vi "FPGAcode.vi"() -> ()   [LabVIEW 2015]
uses:
  <vilib>/Platform/TimedLoop/XDataNode/timing_clust.ctl
  <vilib>/Platform/TimedLoop/XDataNode/nitl_modes.ctl
  <vilib>/Platform/TimedLoop/XDataNode/wakeup.ctl
  <vilib>/rvi/Emulation/niFpgaGetClockAttributes.vi
  <vilib>/rvi/Emulation/niFpgaSctlEmulationGetInTimedLoop.vi
  <vilib>/rvi/Emulation/niFpgaEmulationReportErrorSimple.vi
  <vilib>/rvi/Emulation/niFpgaProcessEmulError.vi
  <vilib>/rvi/eio/common/nirviEmuTemplateMethod_errors.vi
  <vilib>/rvi/Emulation/niFpgaCriticalErrorInLSC.vi
  <vilib>/eio/EIONode/EIONode.xnode
  <vilib>/Platform/TimedLoop/XDataNode/XDataNode.xnode
  <vilib>/Platform/TimedLoop/XDataNode/XDNodeRunTimeDep.lvlib
panel:
  in  "User Command Commit":bool
  in  "User Command":u8
  out "User Command Idle":bool
  out "User Command Status":u8
  in  "User Data 0":u8
  in  "User Data 1":u8
  out "PLL Locked":bool
  out "Filter 1 Detector 3 Correlation":i32
  in  "Filter 2 threshold":i32=1000
  out "Filter 2 Detector 3 Correlation":i32
  in  "Filter 1 threshold":i32=1000
  in  "Filter 3 threshold":i32=1000
  out "Filter 3 Detector 3 Correlation":i32
  in  "Filter 4 threshold":i32=1000
  out "Filter 4 Detector 3 Correlation":i32
  in  "Filter 5 threshold":i32
  out "Filter 5 Detector 3 Correlation":i32
  in  "Filter 6 threshold":i32
  out "Filter 6 Detector 3 Correlation":i32
  in  "Filter 7 threshold":i32
  out "Filter 7 Detector 3 Correlation":i32
  out "Plates":bool
  in  "High Charge Limit":i16
  in  "Low Charge Limit":i16
  in  "High Velocity Count":i32
  in  "Low Velocity Count":i32
  in  "High Mass Limit":i64
  in  "Low Mass Limit":i64
  in  "Mult1":fxp<+,16,7>
  out "Delay1":bool
  in  "One Shot":bool
  out "Not Armed?":bool
  in  "Reset One Shot":bool
  out "Del Not Armed?":bool
  out "IO Module\\AI 0":i16
  out "IO Module\\AI 1":i16
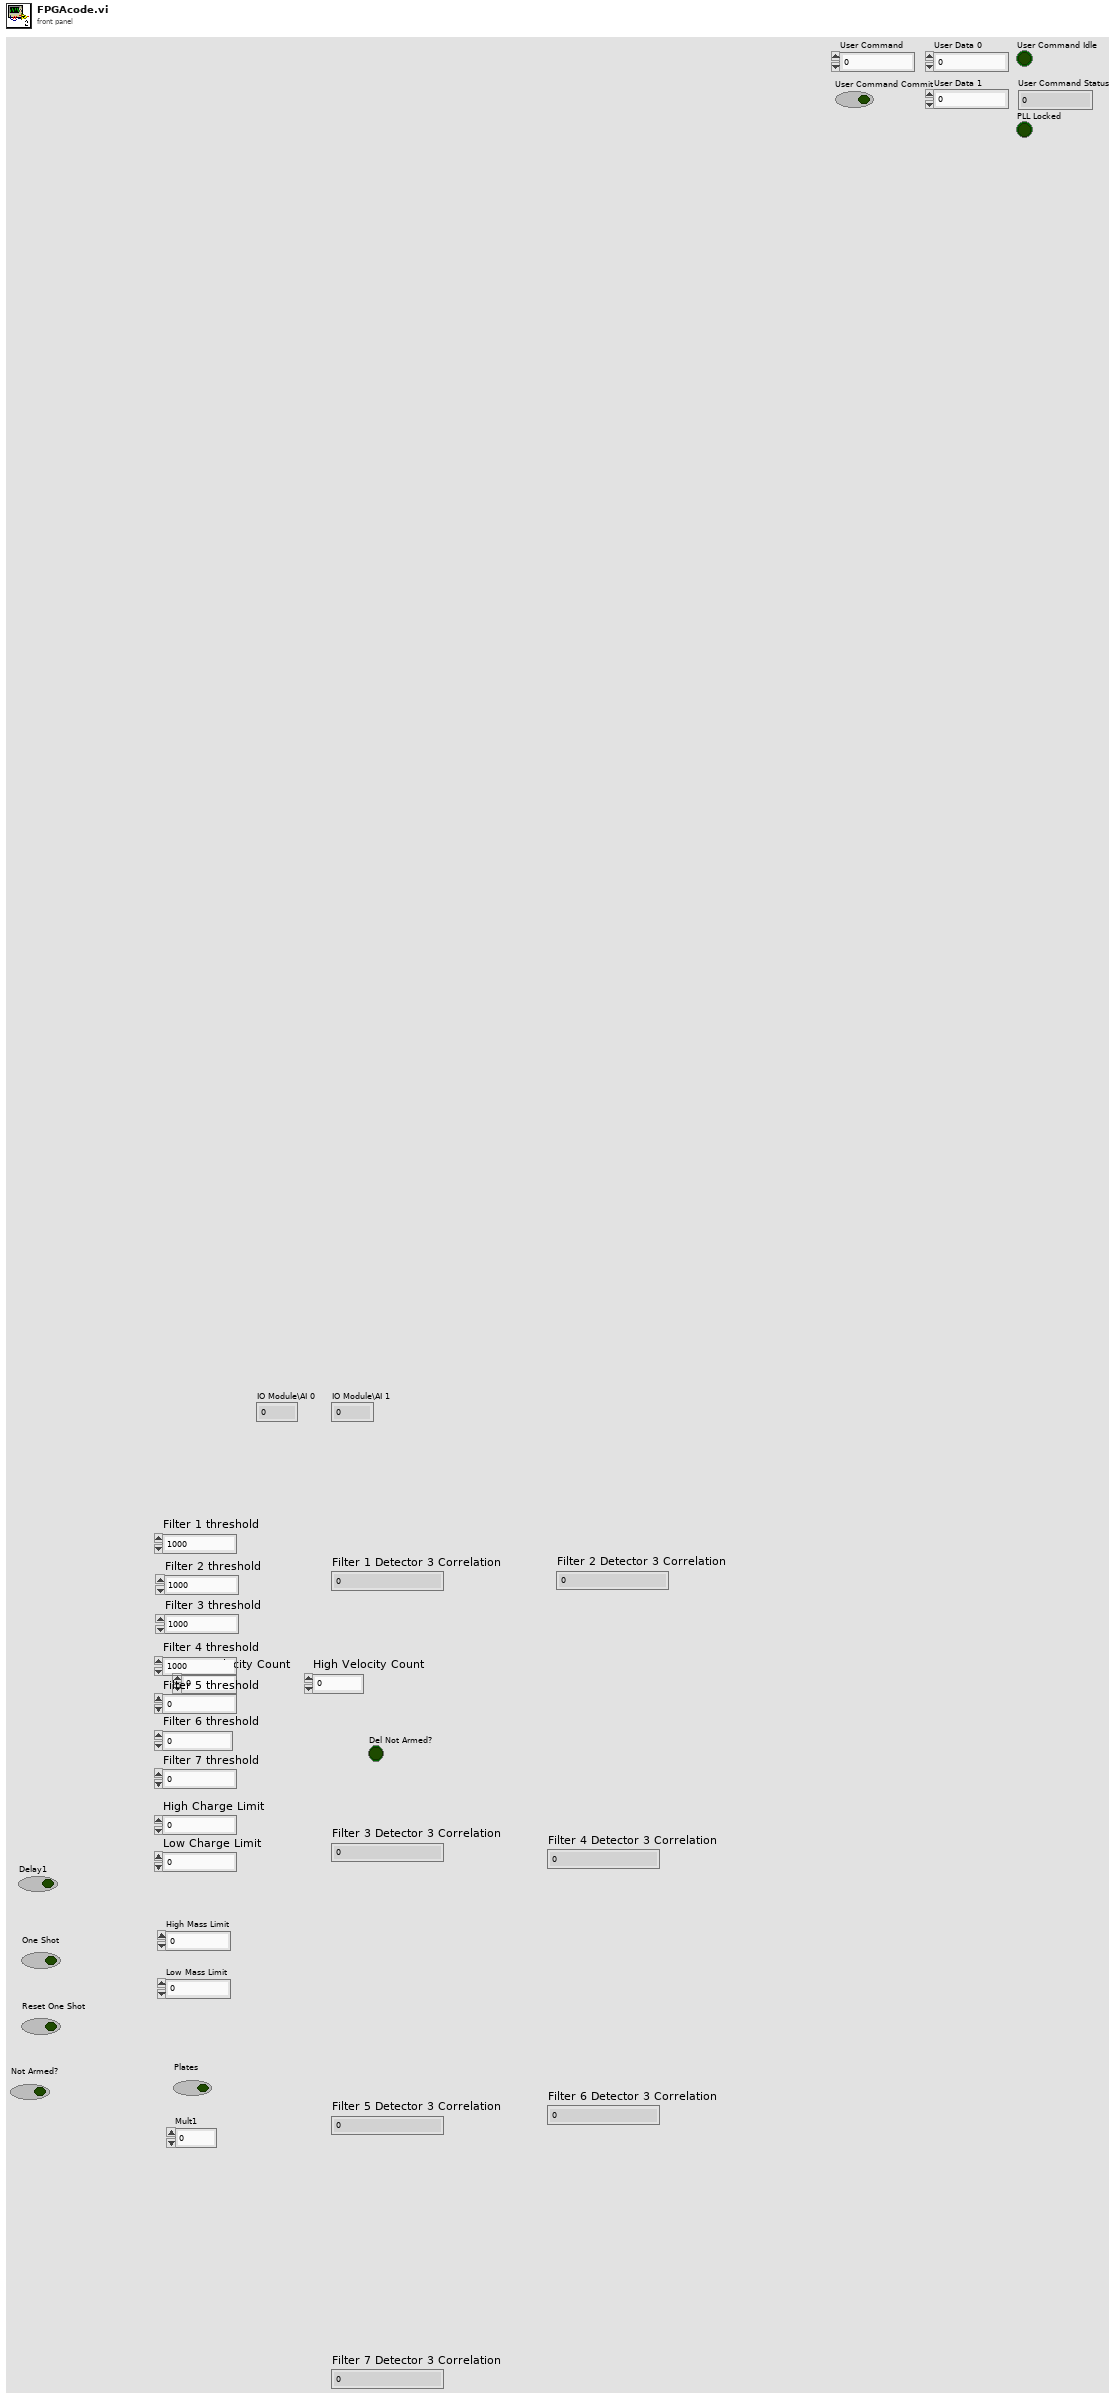
[diagram p1: front panel]
types:
  T1 = typedef "XDNodeRunTimeDep.lvlib/timing_clust.ctl" = cluster{"Expected End [f-1]":u64, "Actual End [f-1]":u64, "Finished Late? [f-1]":bool, "Expected End [i-1]":u64, "Actual End [i-1]":u64, "Finished Late? [i-1]":bool, "Expected Start [i]":u64, "Actual Start [i]":u64, "Expected Start [f]":u64, "Actual Start [f]":u64, "Source Name":string, "Structure Name":string, "Period":i64, "Deadline":i64, "Offset":i64, "Start":i64, "Priority":i32, "Timeout":i32, "Mode":T2, "Wakeup Reason":T3, "Error":errorcluster, "Source Type":string, "Secondary Source Type":string, "Global End Time":u64, "Global Start Time":u64, "Frame Duration":u64, "Iteration Duration":u64, "Assigned CPU":i32, "I/O Scan Engine Mode":u32}
  T2 = typedef "XDNodeRunTimeDep.lvlib/nitl_modes.ctl" = enum32{"No Change", "Process missed periods, maintain original phase", "Discard missed periods, maintain original phase", "Process missed periods, ignore original phase", "Discard missed periods, ignore original phase"}
  T3 = typedef "XDNodeRunTimeDep.lvlib/wakeup.ctl" = enum32{"Normal", "Aborted", "Asynchronous wakeup", "Timing source error", "Timed loop error", "Timeout"}
  T4 = cluster{"Separation cut off 1":i32, "Filter Number":i32, "Separation cut off 2":i32}
  T5 = cluster{"Old Average":i32, "New Average":i32, "Current State":u8, "Detector 1 Correlation":i32, "Detector 3 Correlation":i32, "Velocity Count":i32, "Detector Counter in":i32, "Timeout Count in":i32, "Measured Charge in":i32, "Filter Threshold":i32, "High Correlation in":i32, "Offset":i32, "Offset Average":i32, "Measured Velocity In":i32, "Mult Cluster":cluster{"Mult1":fxp<+,16,7>, "Mult1 Use?":bool}, "Final Delay Count In":u16, "Delay1 In":i32}
  T6 = cluster{"High Charge Limit":i16, "Low Charge Limit":i16, "Low Velocity Count":i32, "High Velocity Count":i32, "Low Velocity Count":i32, fxp<+,30,25>, "High Mass Limit":i64, "Low Mass Limit":i64}
  T7 = cluster{"Average Out":i32, "Next State":u8, "Velocity Count out":i32, "Detector counter out":i32, "Timeout count out":u32, "Measured Charge Out":i32, "High Correlation Out":i32, "Plates":bool, "Offset Out":i32, "Measured Velocity Out":i32, "Final Delay Count Out":u16, "Out1":bool, "Delay1":i32}
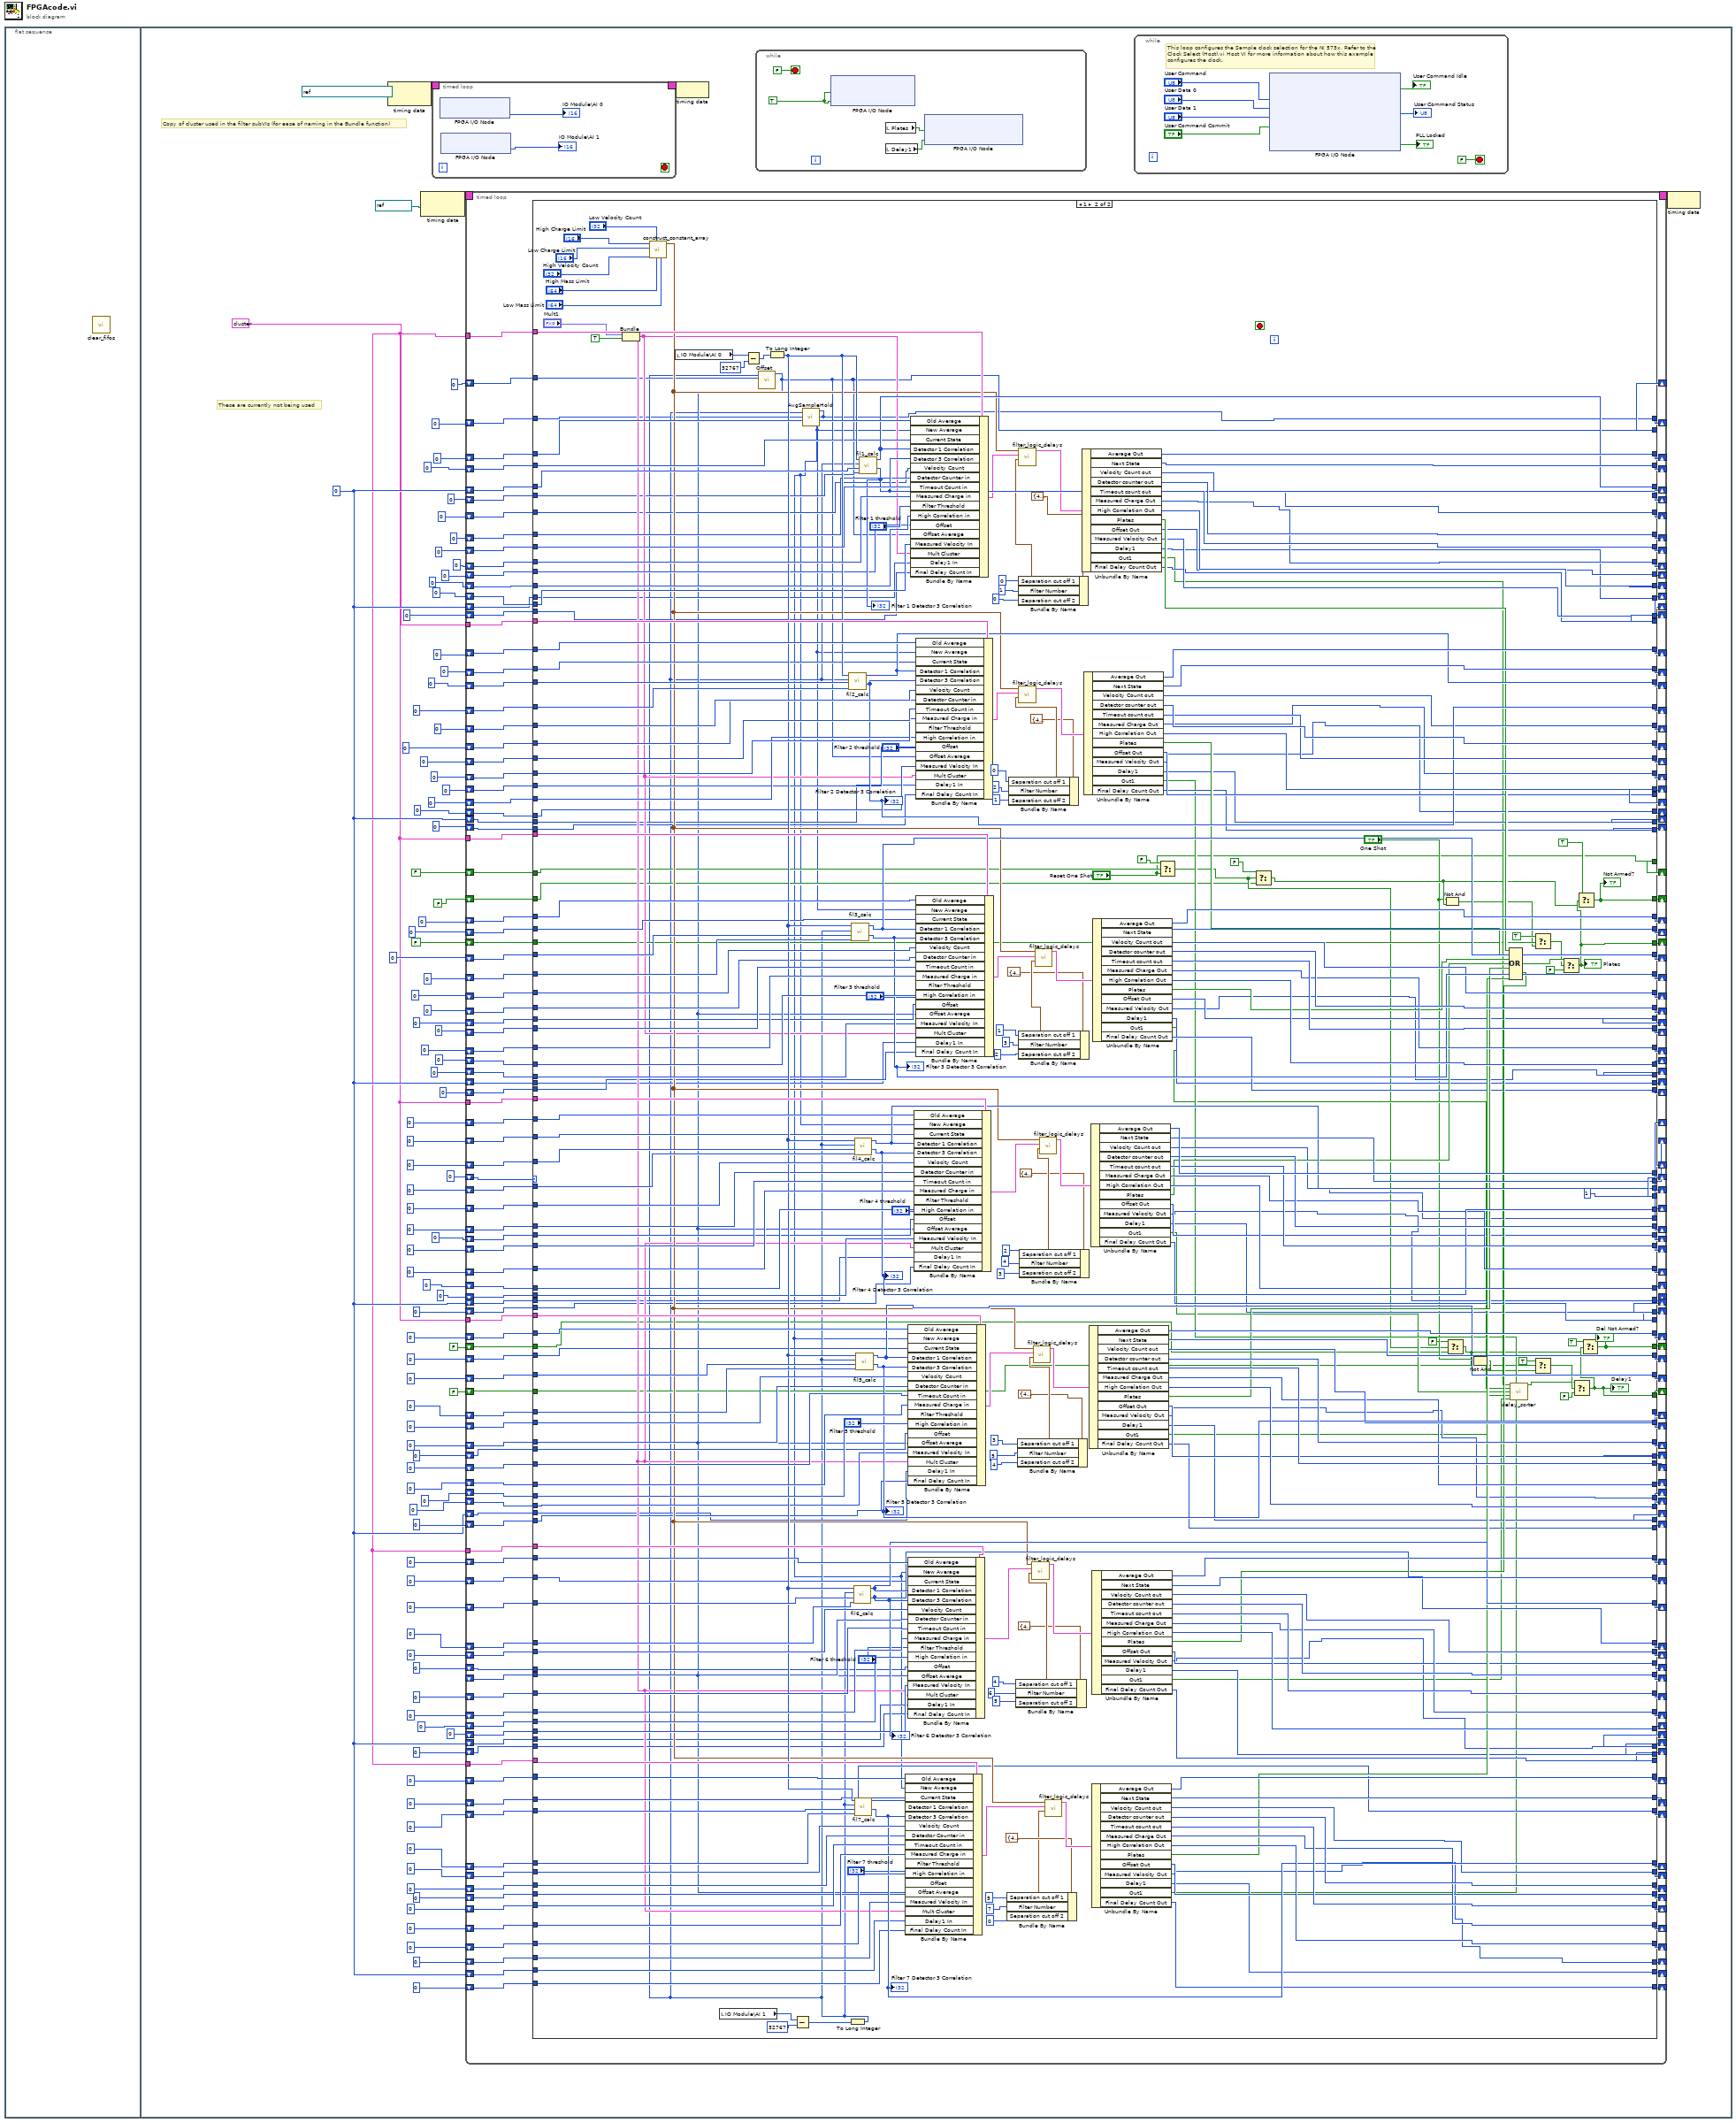
[diagram p0: block diagram]
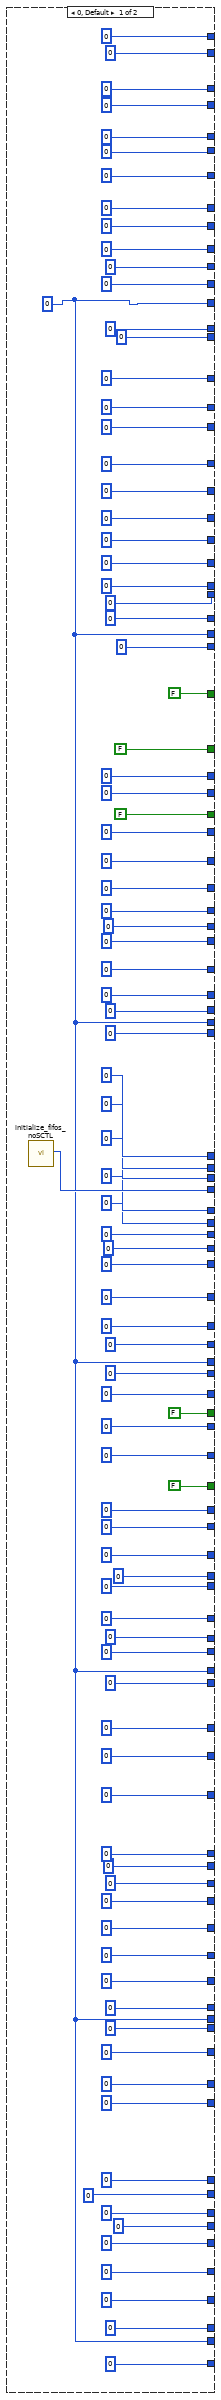
[diagram p2: hidden frame]
diagram:
  n1 = flat-sequence {
    frame #0 {
      n2 = call "clear_fifos.vi"() -> ()  [unwired: 1 in]
    }
    frame #1 {
      w5 = T5 {"Old Average"=0, "New Average"=0, "Current State"=0, "Detector 1 Correlation"=0, "Detector 3 Correlation"=0, "Velocity Count"=0, "Detector Counter in"=0, "Timeout Count in"=0, "Measured Charge in"=0, "Filter Threshold"=0, "High Correlation in"=0, "Offset"=0, "Offset Average"=0, "Measured Velocity In"=0, "Mult Cluster"={"Mult1"=0.0, "Mult1 Use?"=FALSE}, "Final Delay Count In"=0, "Delay1 In"=0} ("Variables Cluster")
      w8 = 0 ("Detector 1 Correlation Out")
      # "These are currently not being used"
      # "Copy of cluster used in the filter subVIs (for ease of naming in the Bundle function)"
      n3 = node-c288(refnum<k21> "IO Module\\Sample Clock" ("Source Name")) -> (w34:T1)
      n4 = node-c288(refnum<k21> "26MHz" ("Source Name")) -> (w98:T1)
      n5 = timed-loop {
        timing: w34 -> [_]
        timing-out: [_] -> w33
        stop <- _ stop-if-true
        n6 = xnode "FPGA I/O Node"() -> ("IO Module\\AI 1"=→"IO Module\\AI 0":u16)  [unwired: 1 in, 1 out]
        n7 = xnode "FPGA I/O Node"() -> ("IO Module\\AI 2"=→"IO Module\\AI 1":u16)  [unwired: 1 in, 1 out]
      }
      n8 = timed-loop {
        timing: w98 -> [_]
        timing-out: [_] -> w97
        shift-right: [w316] -> _
        shift-left: 0 ("Velocity Count out") -> [w238]
        shift-right: [w317] -> _
        shift-left: 0 ("Detector 1 Correlation out") -> [w239]
        shift-right: [w203] -> _
        shift-left: 0 ("Detector counter out") -> [w240]
        shift-right: [w234] -> _
        shift-left: 0 ("Next State") -> [w241]
        shift-right: [w202] -> _
        shift-left: 0 ("Detector 3 Correlation out") -> [w237]
        shift-right: [w315] -> _
        shift-left: 0 ("Timeout count out") -> [w236]
        shift-right: [w230] -> _
        shift-left: 0 ("Next State") -> [w233]
        shift-right: [w229] -> _
        shift-left: 0 ("Detector counter out") -> [w232]
        shift-right: [w201] -> _
        shift-left: 0 ("Detector 1 Correlation out") -> [w309]
        shift-right: [w306] -> _
        shift-left: 0 ("Velocity Count out") -> [w308]
        shift-right: [w305] -> _
        shift-left: u32 0 ("Detector 3 Correlation out") -> [w307]
        shift-right: [w300] -> _
        shift-left: 0 ("Timeout count out") -> [w301]
        shift-right: [w224] -> _
        shift-left: 0 ("Next State") -> [w227]
        shift-right: [w199] -> _
        shift-left: 0 ("Detector counter out") -> [w297]
        shift-right: [w295] -> _
        shift-left: 0 ("Detector 1 Correlation out") -> [w296]
        shift-right: [w293] -> _
        shift-left: u32 0 ("Velocity Count out") -> [w294]
        shift-right: [w198] -> _
        shift-left: 0 ("Detector 3 Correlation out") -> [w292]
        shift-right: [w291] -> _
        shift-left: 0 ("Timeout count out") -> [w226]
        shift-right: [w318] -> _
        shift-left: u8 0 ("High Correlation Out") -> [w321]
        shift-right: [w310] -> _
        shift-left: u8 0 ("High Correlation Out") -> [w311]
        shift-right: [w225] -> _
        shift-left: 0 ("High Correlation Out") -> [w228]
        shift-right: [w319] -> _
        shift-left: 0 ("Measured Charge Out") -> [w322]
        shift-right: [w312] -> _
        shift-left: 0 ("Measured Charge Out") -> [w313]
        shift-right: [w299] -> _
        shift-left: u8 0 ("Measured Charge Out") -> [w298]
        shift-right: [w189] -> _
        shift-left: 0 ("Output New Average") -> [w323]
        shift-right: [w235] -> _
        shift-left: w8 -> [w242]
        tunnel: w5 -> [w320]
        shift-right: [w200] -> _
        shift-left: 0 ("High Sample Out") -> [w303]
        shift-right: [w304] -> _
        shift-left: 0 ("High Correlation Out") -> [w231]
        tunnel: w5 -> [w314]
        tunnel: w5 -> [w302]
        shift-right: [w290] -> _
        shift-left: 0 ("Average Out") -> [w289]
        shift-right: [w288] -> _
        shift-left: u8 0 ("Next State") -> [w287]
        shift-right: [w220] -> _
        shift-left: 0 ("Detector 1 Correlation out") -> [w222]
        shift-right: [w219] -> _
        shift-left: 0 ("Detector 3 Correlation out") -> [w221]
        shift-right: [w197] -> _
        shift-left: 0 ("Velocity Count out") -> [w286]
        shift-right: [w285] -> _
        shift-left: 0 ("Detector counter out") -> [w284]
        shift-right: [w283] -> _
        shift-left: u32 0 ("Timeout count out") -> [w282]
        shift-right: [w196] -> _
        shift-left: 0 ("Measured Charge Out") -> [w281]
        shift-right: [w280] -> _
        shift-left: 0 ("High Correlation Out") -> [w223]
        tunnel: w5 -> [w279]
        shift-right: [w277] -> _
        shift-left: 0 ("Average Out") -> [w276]
        shift-right: [w275] -> _
        shift-left: u8 0 ("Next State") -> [w274]
        shift-right: [w215] -> _
        shift-left: 0 ("Detector 1 Correlation out") -> [w218]
        shift-right: [w214] -> _
        shift-left: 0 ("Detector 3 Correlation out") -> [w217]
        shift-right: [w195] -> _
        shift-left: 0 ("Velocity Count out") -> [w273]
        shift-right: [w272] -> _
        shift-left: 0 ("Detector counter out") -> [w271]
        shift-right: [w270] -> _
        shift-left: u32 0 ("Timeout count out") -> [w269]
        shift-right: [w194] -> _
        shift-left: 0 ("Measured Charge Out") -> [w268]
        shift-right: [w267] -> _
        shift-left: 0 ("High Correlation Out") -> [w216]
        tunnel: w5 -> [w278]
        shift-right: [w265] -> _
        shift-left: 0 ("Average Out") -> [w263]
        shift-right: [w264] -> _
        shift-left: u8 0 ("Next State") -> [w260]
        shift-right: [w210] -> _
        shift-left: 0 ("Detector 1 Correlation out") -> [w213]
        shift-right: [w209] -> _
        shift-left: 0 ("Detector 3 Correlation out") -> [w212]
        shift-right: [w192] -> _
        shift-left: 0 ("Velocity Count out") -> [w262]
        shift-right: [w259] -> _
        shift-left: _ -> [w261]
        shift-right: [w258] -> _
        shift-left: u32 0 ("Timeout count out") -> [w257]
        shift-right: [w193] -> _
        shift-left: 0 ("Measured Charge Out") -> [w256]
        shift-right: [w255] -> _
        shift-left: 0 ("High Correlation Out") -> [w211]
        tunnel: w5 -> [w266]
        shift-right: [w253] -> _
        shift-left: 0 ("Average Out") -> [w252]
        shift-right: [w251] -> _
        shift-left: u8 0 ("Next State") -> [w243]
        shift-right: [w205] -> _
        shift-left: 0 ("Detector 1 Correlation out") -> [w208]
        shift-right: [w204] -> _
        shift-left: 0 ("Detector 3 Correlation out") -> [w207]
        shift-right: [w191] -> _
        shift-left: 0 ("Velocity Count out") -> [w250]
        shift-right: [w249] -> _
        shift-left: 0 ("Detector counter out") -> [w248]
        shift-right: [w247] -> _
        shift-left: u32 0 ("Timeout count out") -> [w246]
        shift-right: [w190] -> _
        shift-left: 0 ("Measured Charge Out") -> [w245]
        shift-right: [w244] -> _
        shift-left: 0 ("High Correlation Out") -> [w206]
        tunnel: w5 -> [w254]
        shift-right: [w187] -> _
        shift-left: i16 0 -> [w188]
        shift-right: [w185] -> _
        shift-left: 0 -> [w186]
        shift-right: [w184] -> _
        shift-left: 0 -> [w181]
        shift-right: [w182] -> _
        shift-left: 0 -> [w183]
        shift-right: [w179] -> _
        shift-left: 0 ("Offset Out") -> [w180]
        shift-right: [w178] -> _
        shift-left: 0 ("Offset Out") -> [w177]
        shift-right: [w176] -> _
        shift-left: 0 ("Offset Out") -> [w175]
        shift-right: [w174] -> _
        shift-left: 0 ("Offset Out") -> [w173]
        shift-right: [w172] -> _
        shift-left: 0 ("Offset Out") -> [w171]
        shift-right: [w169] -> _
        shift-left: 0 -> [w170]
        shift-right: [w168] -> _
        shift-left: 0 -> [w157]
        shift-right: [w167] -> _
        shift-left: 0 -> [w158]
        shift-right: [w166] -> _
        shift-left: 0 -> [w159]
        shift-right: [w165] -> _
        shift-left: 0 -> [w160]
        shift-right: [w164] -> _
        shift-left: 0 -> [w161]
        shift-right: [w163] -> _
        shift-left: 0 ("Measured Velocity Out") -> [w162]
        shift-right: [w156] -> _
        shift-left: w8 -> [w154]
        shift-right: [w155] -> _
        shift-left: u32 0 ("Final Delay Count Out") -> [w153]
        shift-right: [w152] -> _
        shift-left: w8 -> [w150]
        shift-right: [w151] -> _
        shift-left: u32 0 ("Final Delay Count Out") -> [w149]
        shift-right: [w148] -> _
        shift-left: w8 -> [w146]
        shift-right: [w147] -> _
        shift-left: u32 0 ("Final Delay Count Out") -> [w145]
        shift-right: [w144] -> _
        shift-left: w8 -> [w142]
        shift-right: [w143] -> _
        shift-left: u32 0 ("Final Delay Count Out") -> [w141]
        shift-right: [w140] -> _
        shift-left: w8 -> [w138]
        shift-right: [w139] -> _
        shift-left: u32 0 ("Final Delay Count Out") -> [w137]
        shift-right: [w136] -> _
        shift-left: w8 -> [w134]
        shift-right: [w135] -> _
        shift-left: u32 0 ("Final Delay Count Out") -> [w133]
        shift-right: [w132] -> _
        shift-left: w8 -> [w130]
        shift-right: [w131] -> _
        shift-left: u32 0 ("Final Delay Count Out") -> [w129]
        shift-right: [w127] -> _
        shift-left: FALSE -> [w128]
        shift-right: [w126] -> _
        shift-left: FALSE ("f") -> [w125]
        shift-right: [w124] -> _
        shift-left: FALSE ("Reset One Shot") -> [w123]
        shift-right: [w119] -> _
        shift-left: FALSE -> [w122]
        shift-right: [w120] -> _
        shift-left: FALSE -> [w121]
        stop <- _ stop-if-true
        n9 = case shown="1" w188 {
          tunnel: w323 -> [_ w424]
          tunnel: w322 -> [_ w727]
          tunnel: w321 -> [_ w562]
          tunnel: w320 -> [_ w726]
          tunnel: [0 ("Average Out") w725] -> w319
          tunnel: [u16 0 ("Next State") w724] -> w318
          tunnel: [0 ("Detector counter out") w723] -> w317
          tunnel: [u32 0 ("Timeout count out") w722] -> w316
          tunnel: [0 ("High Correlation Out") w721] -> w315
          tunnel: w314 -> [_ w720]
          tunnel: w313 -> [_ w719]
          tunnel: [0 ("Average Out") w718] -> w312
          tunnel: w311 -> [_ w561]
          tunnel: [u16 0 ("Next State") w717] -> w310
          tunnel: w309 -> [_ w716]
          tunnel: w308 -> [_ w554]
          tunnel: w307 -> [_ w715]
          tunnel: [0 ("Detector counter out") w714] -> w306
          tunnel: [u32 0 ("Timeout count out") w713] -> w305
          tunnel: [0 ("High Correlation Out") w712] -> w304
          tunnel: w303 -> [_ w711]
          tunnel: w302 -> [_ w710]
          tunnel: w301 -> [_ w709]
          tunnel: [0 ("Average Out") w708] -> w300
          tunnel: [u16 0 ("Next State") w707] -> w299
          tunnel: w298 -> [_ w560]
          tunnel: w297 -> [_ w706]
          tunnel: w296 -> [_ w553]
          tunnel: [0 ("Detector counter out") w705] -> w295
          tunnel: w294 -> [_ w704]
          tunnel: [u32 0 ("Timeout count out") w703] -> w293
          tunnel: w292 -> [_ w702]
          tunnel: [0 ("High Correlation Out") w701] -> w291
          tunnel: [0 ("Average Out") w700] -> w290
          tunnel: w289 -> [_ w699]
          tunnel: [u16 0 ("Next State") w698] -> w288
          tunnel: w287 -> [_ w559]
          tunnel: w286 -> [_ w697]
          tunnel: [0 ("Detector counter out") w696] -> w285
          tunnel: w284 -> [_ w552]
          tunnel: [u32 0 ("Timeout count out") w695] -> w283
          tunnel: w282 -> [_ w694]
          tunnel: w281 -> [_ w693]
          tunnel: [0 ("High Correlation Out") w692] -> w280
          tunnel: w279 -> [_ w691]
          tunnel: w278 -> [_ w690]
          tunnel: [0 ("Average Out") w689] -> w277
          tunnel: w276 -> [_ w688]
          tunnel: [u16 0 ("Next State") w687] -> w275
          tunnel: w274 -> [_ w558]
          tunnel: w273 -> [_ w686]
          tunnel: [0 ("Detector counter out") w685] -> w272
          tunnel: w271 -> [_ w551]
          tunnel: [u32 0 ("Timeout count out") w684] -> w270
          tunnel: w269 -> [_ w683]
          tunnel: w268 -> [_ w682]
          tunnel: [0 ("High Correlation Out") w681] -> w267
          tunnel: w266 -> [_ w680]
          tunnel: [0 ("Average Out") w679] -> w265
          tunnel: [u16 0 ("Next State") w678] -> w264
          tunnel: w263 -> [_ w677]
          tunnel: w262 -> [_ w676]
          tunnel: w261 -> [_ w550]
          tunnel: w260 -> [_ w557]
          tunnel: [0 ("Detector counter out") w675] -> w259
          tunnel: [u32 0 ("Timeout count out") w674] -> w258
          tunnel: w257 -> [_ w673]
          tunnel: w256 -> [_ w672]
          tunnel: [0 ("High Correlation Out") w671] -> w255
          tunnel: w254 -> [_ w670]
          tunnel: [0 ("Average Out") w669] -> w253
          tunnel: w252 -> [_ w668]
          tunnel: [u16 0 ("Next State") w667] -> w251
          tunnel: w250 -> [_ w666]
          tunnel: [0 ("Detector counter out") w665] -> w249
          tunnel: w248 -> [_ w549]
          tunnel: [u32 0 ("Timeout count out") w664] -> w247
          tunnel: w246 -> [_ w663]
          tunnel: w245 -> [_ w662]
          tunnel: [0 ("High Correlation Out") w661] -> w244
          tunnel: w243 -> [_ w556]
          tunnel: w242 -> [_ w660]
          tunnel: w241 -> [_ w463]
          tunnel: w240 -> [_ w464]
          tunnel: w239 -> [_ w555]
          tunnel: w238 -> [_ w659]
          tunnel: w237 -> [_ w658]
          tunnel: w236 -> [_ w657]
          tunnel: [0 ("Detector 1 Correlation Out") w656] -> w235
          tunnel: [0 ("Detector 3 Correlation Out") w655] -> w234
          tunnel: w233 -> [_ w654]
          tunnel: w232 -> [_ w653]
          tunnel: w231 -> [_ w652]
          tunnel: [0 ("Detector 1 Correlation Out") w651] -> w230
          tunnel: [0 ("Detector 3 Correlation Out") w650] -> w229
          tunnel: w228 -> [_ w649]
          tunnel: w227 -> [_ w648]
          tunnel: w226 -> [_ w647]
          tunnel: [0 ("Detector 1 Correlation Out") w646] -> w225
          tunnel: [0 ("Detector 3 Correlation Out") w645] -> w224
          tunnel: w223 -> [_ w644]
          tunnel: w222 -> [_ w643]
          tunnel: w221 -> [_ w642]
          tunnel: [0 ("Detector 1 Correlation Out") w641] -> w220
          tunnel: [0 ("Detector 3 Correlation Out") w640] -> w219
          tunnel: w218 -> [_ w639]
          tunnel: w217 -> [_ w638]
          tunnel: w216 -> [_ w637]
          tunnel: [0 ("Detector 1 Correlation Out") w636] -> w215
          tunnel: [0 ("Detector 3 Correlation Out") w635] -> w214
          tunnel: w213 -> [_ w634]
          tunnel: w212 -> [_ w633]
          tunnel: w211 -> [_ w632]
          tunnel: [0 ("Detector 1 Correlation Out") w631] -> w210
          tunnel: [0 ("Detector 3 Correlation Out") w630] -> w209
          tunnel: w208 -> [_ w629]
          tunnel: w207 -> [_ w628]
          tunnel: w206 -> [_ w627]
          tunnel: [0 ("Detector 1 Correlation Out") w498] -> w205
          tunnel: [0 ("Detector 3 Correlation Out") w626] -> w204
          tunnel: [0 ("Velocity Count out") w625] -> w203
          tunnel: [0 ("Measured Charge Out") w624] -> w202
          tunnel: [0 ("Velocity Count out") w623] -> w201
          tunnel: [0 ("Measured Charge Out") w622] -> w200
          tunnel: [0 ("Velocity Count out") w621] -> w199
          tunnel: [0 ("Measured Charge Out") w620] -> w198
          tunnel: [0 ("Velocity Count out") w548] -> w197
          tunnel: [0 ("Measured Charge Out") w619] -> w196
          tunnel: [0 ("Velocity Count out") w618] -> w195
          tunnel: [0 ("Measured Charge Out") w617] -> w194
          tunnel: [0 ("Measured Charge Out") w616] -> w193
          tunnel: [0 ("Velocity Count out") w615] -> w192
          tunnel: [0 ("Velocity Count out") w614] -> w191
          tunnel: [0 ("Measured Charge Out") w613] -> w190
          tunnel: [0 ("Output New Average") w423] -> w189
          tunnel: [w416 i16 1 ("Output State")] -> w187
          tunnel: w186 -> [_ w547]
          tunnel: [0 ("Offset Out") w546] -> w185
          tunnel: [0 ("Offset Out") w545] -> w184
          tunnel: w183 -> [_ w427]
          tunnel: [0 ("Output New Average") w426] -> w182
          tunnel: w181 -> [_ w544]
          tunnel: w180 -> [_ w543]
          tunnel: [0 ("Offset Out") w542] -> w179
          tunnel: [0 ("Offset Out") w541] -> w178
          tunnel: w177 -> [_ w540]
          tunnel: [0 ("Offset Out") w539] -> w176
          tunnel: w175 -> [_ w538]
          tunnel: [0 ("Offset Out") w537] -> w174
          tunnel: w173 -> [_ w536]
          tunnel: [0 ("Offset Out") w535] -> w172
          tunnel: w171 -> [_ w534]
          tunnel: w170 -> [_ w529]
          tunnel: [0 ("Measured Velocity Out") w522] -> w169
          tunnel: [0 ("Measured Velocity Out") w521] -> w168
          tunnel: [0 ("Measured Velocity Out") w520] -> w167
          tunnel: [0 ("Measured Velocity Out") w519] -> w166
          tunnel: [0 ("Measured Velocity Out") w518] -> w165
          tunnel: [0 ("Measured Velocity Out") w517] -> w164
          tunnel: [0 ("Measured Velocity Out") w516] -> w163
          tunnel: w162 -> [_ w528]
          tunnel: w161 -> [_ w527]
          tunnel: w160 -> [_ w526]
          tunnel: w159 -> [_ w525]
          tunnel: w158 -> [_ w524]
          tunnel: w157 -> [_ w523]
          tunnel: [w329 w493] -> w156
          tunnel: [u32 0 ("Final Delay Count Out") w511] -> w155
          tunnel: w154 -> [_ w510]
          tunnel: w153 -> [_ w509]
          tunnel: [w329 w508] -> w152
          tunnel: [u32 0 ("Final Delay Count Out") w507] -> w151
          tunnel: w150 -> [_ w506]
          tunnel: w149 -> [_ w505]
          tunnel: [w329 w492] -> w148
          tunnel: [u32 0 ("Final Delay Count Out") w504] -> w147
          tunnel: w146 -> [_ w485]
          tunnel: w145 -> [_ w503]
          tunnel: [w329 w491] -> w144
          tunnel: [u32 0 ("Final Delay Count Out") w502] -> w143
          tunnel: w142 -> [_ w484]
          tunnel: w141 -> [_ w501]
          tunnel: [w329 w490] -> w140
          tunnel: [u32 0 ("Final Delay Count Out") w500] -> w139
          tunnel: w138 -> [_ w483]
          tunnel: w137 -> [_ w499]
          tunnel: [w329 w489] -> w136
          tunnel: [u32 0 ("Final Delay Count Out") w497] -> w135
          tunnel: w134 -> [_ w482]
          tunnel: w133 -> [_ w496]
          tunnel: [w329 w488] -> w132
          tunnel: [u32 0 ("Final Delay Count Out") w495] -> w131
          tunnel: w130 -> [_ w481]
          tunnel: w129 -> [_ w494]
          tunnel: w128 -> [_ w429]
          tunnel: [FALSE ("t") w449] -> w127
          tunnel: [FALSE ("f") w461] -> w126
          tunnel: w125 -> [_ w460]
          tunnel: [FALSE ("Reset One Shot") "Reset One Shot"] -> w124
          tunnel: w123 -> [_ w447]
          tunnel: w122 -> [_ w430]
          tunnel: w121 -> [_ w436]
          tunnel: [FALSE ("Delay1") w435] -> w120
          tunnel: [FALSE w432] -> w119
          frame 0, Default {
            w329 = 0
            n10 = call "initialize_fifos_noSCTL.vi"() -> ("Output State"=w416:i16)  [unwired: 11 in]
          }
          frame 1 {
            n11 = Bundle("Mult1"="Mult1", TRUE) -> (w512:cluster{"Mult1":fxp<+,16,7>, bool})  [unwired: 1 in]
            n12 = call "construct_constant_array.vi"("Low Mass Limit"="Low Mass Limit", "High Mass Limit"="High Mass Limit", "Low Velocity Count"="Low Velocity Count", "High Velocity Count"="High Velocity Count", "Low Charge Limit"="Low Charge Limit", "High Charge Limit"="High Charge Limit") -> ("constants cluster"=w513:T6)  [unwired: 5 in]
            n13 = local read "IO Module\\AI 0"() -> (w422:i16)
            n14 = local read "IO Module\\AI 1"() -> (w419:i16)
            n15 = Subtract(x=w422, y=i16 32767) -> (x-y=w420:i16)
            n16 = To Long Integer(number=w420) -> (32bit integer=w571:i32)
            n17 = Subtract(x=w419, y=i16 32767) -> (x-y=w417:i16)
            n18 = To Long Integer(number=w417) -> (32bit integer=w425:i32)
            n19 = call "Offset.vi"("Previous Average"=w427, "Input Value"=w425) -> ("Output New Average"=w426:i32)  [unwired: 9 in]
            n20 = call "AvgSampleHold.vi"("Previous Average"=w424, "Input Value"=w425) -> ("Output New Average"=w423:i32)  [unwired: 9 in]
            n21 = call "fil2_calc.vi"("Detector 3 Correlation In"=w653, "Detector 1 Correlation In"=w654, "AI1"=w425, "AI0"=w571) -> ("Detector 3 Correlation Out"=w650:i32, "Detector 1 Correlation Out"=w651:i32)  [unwired: 4 in]
            "Filter 2 Detector 3 Correlation" <- w650
            n22 = call "fil3_calc.vi"("Detector 3 Correlation In"=w648, "Detector 1 Correlation In"=w649, "AI1"=w425, "AI0"=w571) -> ("Detector 3 Correlation Out"=w645:i32, "Detector 1 Correlation Out"=w646:i32)  [unwired: 4 in]
            "Filter 3 Detector 3 Correlation" <- w645
            n23 = call "fil6_calc.vi"("Detector 3 Correlation In"=w633, "Detector 1 Correlation In"=w634, "AI1"=w425, "AI0"=w571) -> ("Detector 3 Correlation Out"=w630:i32, "Detector 1 Correlation Out"=w631:i32)  [unwired: 4 in]
            "Filter 6 Detector 3 Correlation" <- w630
            n24 = call "fil4_calc.vi"("Detector 3 Correlation In"=w642, "Detector 1 Correlation In"=w643, "AI1"=w425, "AI0"=w571) -> ("Detector 3 Correlation Out"=w640:i32, "Detector 1 Correlation Out"=w641:i32)  [unwired: 4 in]
            "Filter 4 Detector 3 Correlation" <- w640
            n25 = call "fil7_calc.vi"("Detector 3 Correlation In"=w628, "Detector 1 Correlation In"=w629, "AI1"=w425, "AI0"=w571) -> ("Detector 3 Correlation Out"=w626:i32, "Detector 1 Correlation Out"=w498:i32)  [unwired: 4 in]
            "Filter 7 Detector 3 Correlation" <- w626
            n26 = call "fil5_calc.vi"("Detector 3 Correlation In"=w638, "Detector 1 Correlation In"=w639, "AI1"=w425, "AI0"=w571) -> ("Detector 3 Correlation Out"=w635:i32, "Detector 1 Correlation Out"=w636:i32)  [unwired: 4 in]
            "Filter 5 Detector 3 Correlation" <- w635
            n27 = call "fil1_calc.vi"("Detector 3 Correlation In"=w463, "Detector 1 Correlation In"=w660, "AI1"=w425, "AI0"=w571) -> ("Detector 3 Correlation Out"=w655:i32, "Detector 1 Correlation Out"=w656:i32)  [unwired: 4 in]
            "Filter 1 Detector 3 Correlation" <- w655
            n28 = Bundle By Name(cluster=w670, "Old Average"=w668, "New Average"=w423, "Current State"=w556, "Detector 1 Correlation"=w498, "Detector 3 Correlation"=w626, "Velocity Count"=w666, "Detector Counter in"=w549, "Timeout Count in"=w663, "Measured Charge in"=w662, "Filter Threshold"="Filter 7 threshold", "High Correlation in"=w627, "Offset"=w534, "Offset Average"=w426, "Measured Velocity In"=w528, "Mult Cluster"=w512, "Delay1 In"=w481, "Final Delay Count In"=w494) -> (w451:T5)
            n29 = Bundle By Name(cluster=w680, "Old Average"=w677, "New Average"=w423, "Current State"=w557, "Detector 1 Correlation"=w631, "Detector 3 Correlation"=w630, "Velocity Count"=w676, "Detector Counter in"=w550, "Timeout Count in"=w673, "Measured Charge in"=w672, "Filter Threshold"="Filter 6 threshold", "High Correlation in"=w632, "Offset"=w536, "Offset Average"=w426, "Measured Velocity In"=w527, "Mult Cluster"=w512, "Delay1 In"=w482, "Final Delay Count In"=w496) -> (w452:T5)
            n30 = Bundle By Name(cluster=w690, "Old Average"=w688, "New Average"=w423, "Current State"=w558, "Detector 1 Correlation"=w636, "Detector 3 Correlation"=w635, "Velocity Count"=w686, "Detector Counter in"=w551, "Timeout Count in"=w683, "Measured Charge in"=w682, "Filter Threshold"="Filter 5 threshold", "High Correlation in"=w637, "Offset"=w538, "Offset Average"=w426, "Measured Velocity In"=w526, "Mult Cluster"=w512, "Delay1 In"=w483, "Final Delay Count In"=w499) -> (w453:T5)
            n31 = Bundle By Name(cluster=w726, "Old Average"=w727, "New Average"=w423, "Current State"=w562, "Detector 1 Correlation"=w656, "Detector 3 Correlation"=w655, "Velocity Count"=w464, "Detector Counter in"=w555, "Timeout Count in"=w659, "Measured Charge in"=w658, "Filter Threshold"="Filter 1 threshold", "High Correlation in"=w657, "Offset"=w547, "Offset Average"=w426, "Measured Velocity In"=w529, "Mult Cluster"=w512, "Delay1 In"=w510, "Final Delay Count In"=w509) -> (w457:T5)
            n32 = Bundle By Name(cluster=w691, "Old Average"=w699, "New Average"=w423, "Current State"=w559, "Detector 1 Correlation"=w641, "Detector 3 Correlation"=w640, "Velocity Count"=w697, "Detector Counter in"=w552, "Timeout Count in"=w694, "Measured Charge in"=w693, "Filter Threshold"="Filter 4 threshold", "High Correlation in"=w644, "Offset"=w540, "Offset Average"=w426, "Measured Velocity In"=w525, "Mult Cluster"=w512, "Delay1 In"=w484, "Final Delay Count In"=w501) -> (w454:T5)
            n33 = Bundle By Name(cluster=w720, "Old Average"=w719, "New Average"=w423, "Current State"=w561, "Detector 1 Correlation"=w651, "Detector 3 Correlation"=w650, "Velocity Count"=w716, "Detector Counter in"=w554, "Timeout Count in"=w715, "Measured Charge in"=w711, "Filter Threshold"="Filter 2 threshold", "High Correlation in"=w652, "Offset"=w544, "Offset Average"=w426, "Measured Velocity In"=w523, "Mult Cluster"=w512, "Delay1 In"=w506, "Final Delay Count In"=w505) -> (w456:T5)
            n34 = Bundle By Name(cluster=w710, "Old Average"=w709, "New Average"=w423, "Current State"=w560, "Detector 1 Correlation"=w646, "Detector 3 Correlation"=w645, "Velocity Count"=w706, "Detector Counter in"=w553, "Timeout Count in"=w704, "Measured Charge in"=w702, "Filter Threshold"="Filter 3 threshold", "High Correlation in"=w647, "Offset"=w543, "Offset Average"=w426, "Measured Velocity In"=w524, "Mult Cluster"=w512, "Delay1 In"=w485, "Final Delay Count In"=w503) -> (w455:T5)
            n35 = Bundle By Name(cluster=T4 {"Separation cut off 1"=4, "Filter Number"=5, "Separation cut off 2"=6} ("Filter Specific Constants"), "Separation cut off 1"=5, "Filter Number"=7, "Separation cut off 2"=0) -> (w467:T4)
            n36 = Bundle By Name(cluster=T4 {"Separation cut off 1"=4, "Filter Number"=5, "Separation cut off 2"=6} ("Filter Specific Constants"), "Separation cut off 1"=0, "Filter Number"=2, "Separation cut off 2"=1) -> (w604:T4)
            n37 = Bundle By Name(cluster=T4 {"Separation cut off 1"=4, "Filter Number"=5, "Separation cut off 2"=6} ("Filter Specific Constants"), "Separation cut off 1"=4, "Filter Number"=6, "Separation cut off 2"=5) -> (w594:T4)
            n38 = Bundle By Name(cluster=T4 {"Separation cut off 1"=4, "Filter Number"=5, "Separation cut off 2"=6} ("Filter Specific Constants"), "Separation cut off 1"=3, "Filter Number"=5, "Separation cut off 2"=4) -> (w596:T4)
            n39 = Bundle By Name(cluster=T4 {"Separation cut off 1"=4, "Filter Number"=5, "Separation cut off 2"=6} ("Filter Specific Constants"), "Separation cut off 1"=0, "Filter Number"=1, "Separation cut off 2"=0) -> (w602:T4)
            n40 = call "filter_logic_delays.vi"("Filter Specific Constants"=w602, "Variables Cluster"=w457, "controls cluster"=w513) -> ("Output Cluster"=w601:T7)  [unwired: 8 in]
            n41 = call "filter_logic_delays.vi"("Filter Specific Constants"=w604, "Variables Cluster"=w456, "controls cluster"=w513) -> ("Output Cluster"=w611:T7)  [unwired: 8 in]
            n42 = Bundle By Name(cluster=T4 {"Separation cut off 1"=4, "Filter Number"=5, "Separation cut off 2"=6} ("Filter Specific Constants"), "Separation cut off 1"=1, "Filter Number"=3, "Separation cut off 2"=2) -> (w600:T4)
            n43 = Bundle By Name(cluster=T4 {"Separation cut off 1"=4, "Filter Number"=5, "Separation cut off 2"=6} ("Filter Specific Constants"), "Separation cut off 1"=2, "Filter Number"=4, "Separation cut off 2"=3) -> (w598:T4)
            n44 = call "filter_logic_delays.vi"("Filter Specific Constants"=w594, "Variables Cluster"=w452, "controls cluster"=w513) -> ("Output Cluster"=w593:T7)  [unwired: 8 in]
            n45 = call "filter_logic_delays.vi"("Filter Specific Constants"=w596, "Variables Cluster"=w453, "controls cluster"=w513) -> ("Output Cluster"=w595:T7)  [unwired: 8 in]
            n46 = call "filter_logic_delays.vi"("Filter Specific Constants"=w600, "Variables Cluster"=w455, "controls cluster"=w513) -> ("Output Cluster"=w599:T7)  [unwired: 8 in]
            n47 = call "filter_logic_delays.vi"("Filter Specific Constants"=w598, "Variables Cluster"=w454, "controls cluster"=w513) -> ("Output Cluster"=w597:T7)  [unwired: 8 in]
            n48 = call "filter_logic_delays.vi"("Filter Specific Constants"=w467, "Variables Cluster"=w451, "controls cluster"=w513) -> ("Output Cluster"=w603:T7)  [unwired: 8 in]
            n49 = Unbundle By Name(w601) -> ("Average Out"=w725:i32, "Next State"=w724:u8, "Velocity Count out"=w625:i32, "Detector counter out"=w723:i32, "Timeout count out"=w722:u32, "Measured Charge Out"=w624:i32, "High Correlation Out"=w721:i32, "Plates"=w569:bool, "Offset Out"=w546:i32, "Measured Velocity Out"=w522:i32, "Delay1"=w493:i32, "Out1"=w487:bool, "Final Delay Count Out"=w511:u16)
            n50 = Unbundle By Name(w611) -> ("Average Out"=w718:i32, "Next State"=w717:u8, "Velocity Count out"=w623:i32, "Detector counter out"=w714:i32, "Timeout count out"=w713:u32, "Measured Charge Out"=w622:i32, "High Correlation Out"=w712:i32, "Plates"=w568:bool, "Offset Out"=w545:i32, "Measured Velocity Out"=w521:i32, "Delay1"=w508:i32, "Out1"=w486:bool, "Final Delay Count Out"=w507:u16)
            n51 = Unbundle By Name(w595) -> ("Average Out"=w689:i32, "Next State"=w687:u8, "Velocity Count out"=w618:i32, "Detector counter out"=w685:i32, "Timeout count out"=w684:u32, "Measured Charge Out"=w617:i32, "High Correlation Out"=w681:i32, "Plates"=w565:bool, "Offset Out"=w539:i32, "Measured Velocity Out"=w518:i32, "Delay1"=w490:i32, "Out1"=w477:bool, "Final Delay Count Out"=w500:u16)
            n52 = Unbundle By Name(w597) -> ("Average Out"=w700:i32, "Next State"=w698:u8, "Velocity Count out"=w548:i32, "Detector counter out"=w696:i32, "Timeout count out"=w695:u32, "Measured Charge Out"=w619:i32, "High Correlation Out"=w692:i32, "Plates"=w566:bool, "Offset Out"=w541:i32, "Measured Velocity Out"=w519:i32, "Delay1"=w491:i32, "Out1"=w478:bool, "Final Delay Count Out"=w502:u16)
            n53 = Unbundle By Name(w603) -> ("Average Out"=w669:i32, "Next State"=w667:u8, "Velocity Count out"=w614:i32, "Detector counter out"=w665:i32, "Timeout count out"=w664:u32, "Measured Charge Out"=w613:i32, "High Correlation Out"=w661:i32, "Plates"=w563:bool, "Offset Out"=w535:i32, "Measured Velocity Out"=w516:i32, "Delay1"=w488:i32, "Out1"=w476:bool, "Final Delay Count Out"=w495:u16)
            n54 = Unbundle By Name(w593) -> ("Average Out"=w679:i32, "Next State"=w678:u8, "Velocity Count out"=w615:i32, "Detector counter out"=w675:i32, "Timeout count out"=w674:u32, "Measured Charge Out"=w616:i32, "High Correlation Out"=w671:i32, "Plates"=w564:bool, "Offset Out"=w537:i32, "Measured Velocity Out"=w517:i32, "Delay1"=w489:i32, "Out1"=w475:bool, "Final Delay Count Out"=w497:u16)
            n55 = Unbundle By Name(w599) -> ("Average Out"=w708:i32, "Next State"=w707:u8, "Velocity Count out"=w621:i32, "Detector counter out"=w705:i32, "Timeout count out"=w703:u32, "Measured Charge Out"=w620:i32, "High Correlation Out"=w701:i32, "Plates"=w567:bool, "Offset Out"=w542:i32, "Measured Velocity Out"=w520:i32, "Delay1"=w492:i32, "Out1"=w479:bool, "Final Delay Count Out"=w504:u16)
            n56 = Select(t=FALSE, s=w447, f="Reset One Shot") -> (s? t:f=w438:bool)
            n57 = Select(t=FALSE, s=w438, f=w429) -> (s? t:f=w450:bool)
            n58 = Not And(1:w450, 2:"One Shot") -> (0:w441:bool)
            n59 = Select(t=FALSE, s=w438, f=w430) -> (s? t:f=w433:bool)
            n60 = Not And(1:w433, 2:"One Shot") -> (0:w439:bool)
            n61 = Compound Arithmetic op=OR(w569, w568, w567, w566, w565, w564, w563) -> (w466:bool)
            n62 = call "delay_sorter.vi"("Out1 1"=w487, "Out1 2"=w486, "Out1 3"=w479, "Out1 4"=w478, "Out1 5"=w477, "Out1 6"=w475, "Out1 7"=w476) -> ("Delay1"=w443:bool)  [unwired: 8 in]
            n63 = Select(t=TRUE, s=w460, f=w441) -> (s? t:f=w458:bool)
            n64 = Select(t=TRUE, s=w436, f=w439) -> (s? t:f=w445:bool)
            n65 = Select(t=w466, s=w458, f=FALSE) -> (s? t:f=w461:bool)
            "Plates" <- w461
            n66 = Select(t=w443, s=w445, f=FALSE) -> (s? t:f=w435:bool)
            "Delay1" <- w435
            n67 = Select(t=TRUE, s=w461, f=w450) -> (s? t:f=w449:bool)
            "Not Armed?" <- w449
            n68 = Select(t=TRUE, s=w435, f=w433) -> (s? t:f=w432:bool)
            "Del Not Armed?" <- w432
          }
        }
      }
      n69 = node-c288(w33) -> ()
      n70 = while {
        stop <- FALSE stop-if-true
        w117 = TRUE ("IO Module\\PFI Enable")
        n71 = xnode "FPGA I/O Node"("IO Module\\PFI 0 WE"=w117, "IO Module\\PFI 1 WE"=w117) -> ()  [unwired: 2 in, 2 out]
        n72 = local read "Plates"() -> (w116:bool)
        n73 = local read "Delay1"() -> (w115:bool)
        n74 = xnode "FPGA I/O Node"("IO Module\\PFI 0 Wr Data"=w116, "IO Module\\PFI 1 Wr Data"=w115) -> ()  [unwired: 2 in, 2 out]
      }
      n75 = while {
        stop <- FALSE stop-if-true
        # "This loop configures the Sample clock selection for the NI 573x. Refer to the Clock Select (Host).vi Host VI for more information about how this example configures the clock."
        n76 = xnode "FPGA I/O Node"("IO Module\\User Command"="User Command", "IO Module\\User Data 0"="User Data 0", "IO Module\\User Data 1"="User Data 1", "IO Module\\User Command Commit"="User Command Commit") -> ("IO Module\\User Command Idle"=→"User Command Idle":bool, "IO Module\\User Command Status"=→"User Command Status":u8, "IO Module\\PLL Locked"=→"PLL Locked":bool)  [unwired: 7 in, 7 out]
      }
      n77 = node-c288(w97) -> ()
    }
  }
